vi "DHE_ParseCommand.vi"(0 "fd":i32, 1 "Log":bool=TRUE, 5 "command + args":string, 7 "command":string, 9 "arguments":string, 11 "error in":errorcluster, 12 "modpath":path) -> (4 "DHE_DBSRef":T1, 6 "message":string, 8 "OK message":string="DONE", 10 "TimeOut out":i32, 15 "error out":errorcluster)   [LabVIEW 2016]
uses:
  DBSHAND/private/vis/DatabaseHand_RefNum.ctl
  DHE_TP_action.ctl
  DBSHAND/private/vis/DatabaseHand_Element_Get(string).vi
  DBSHAND/private/vis/DatabaseHand_Element_Set(double).vi
  DBSHAND/private/vis/DatabaseHand_Element_Get(bool).vi
  DBSHAND/private/vis/DatabaseHand_Element_Get(double).vi
  DBSHAND/private/vis/DatabaseHand_Element_Get(I32).vi
  DBSHAND/private/vis/DatabaseHand_Element_Get(U32).vi
  DBSHAND/private/vis/DatabaseHand_Element_Set(string).vi
  DBSHAND/private/vis/DatabaseHand_Element_Set(2DArr).vi
  DBSHAND/private/vis/DatabaseHand_Element_Set(bool).vi
panel:
  in  "DHE_Aliasfile":path
  out "timeout offset":i32=20000
  in  "initimeout":i32=-1
  out "expscript":path
  in  "shutdownmacro":string
  in  "initmacro":string
  in  "extshut":bool
  in  "appendid":bool
  in  "expasync":bool=TRUE
  in  "artifpatterns":string
  in  "FPAreadmode":string
  in  "FPAmodifiers":string
  in  "FPAname":string
  in  "DHE_InstLib":path
  in  "DHE_REGfile":path
  in  "DHE_DACfile":path
  in  "DHE_Mod":string
  in  "log":bool
  in  "DHE_LogFile":path
  in  "DHE_MacroDir":path
  out "ConfigFile":path
  in  "Algors_file":path
  in  "TP_file":path
  in  "Init_file":path
  in  "Config":string[][](table)=[["INIT", "file", "DHE_ParseCommand.vi", "Init_file", "none", "PATH"], ["INIT", "module", "DHE_ParseCommand.vi", "DHE_Mod", "", "STR"], ["INIT", "initmacro", "DHE_ParseCommand.vi", "initmacro", "", "STR"], ["INIT", "timeout_s", "DHE_ParseCommand.vi", "initimeout", "", "I32"], ["TP", "tpfile", "DHE_ParseCommand.vi", "TP_file", "none", "PATH"], ["TP", "algorfile", "DHE_ParseCommand.vi", "Algors_file", "none", "PATH"], ["LOG", "file", "DHE_ParseCommand.vi", "DHE_LogFile", "none", "PATH"], ["LOG", "log", "DHE_ParseCommand.vi", "log", "FALSE", "BOOL"], ["MACROS", "dir", "DHE_ParseCommand.vi", "DHE_MacroDir", "", "PATH"], ["DACS", "file", "DHE_ParseCommand.vi", "DHE_DACfile", "", "PATH"], ["REGS", "file", "DHE_ParseCommand.vi", "DHE_REGfile", "", "PATH"], ["INSTLIB", "lib", "DHE_ParseCommand.vi", "DHE_InstLib", "", "PATH"], ["FPA", "name", "DHE_ParseCommand.vi", "FPAname", "", "STR"], ["FPA", "modifiers", "DHE_ParseCommand.vi", "FPAmodifiers", "", "STR"], ["FPA", "readmode", "DHE_ParseCommand.vi", "FPAreadmode", "", "STR"], ["ARTIF", "patterns", "DHE_ParseCommand.vi", "artifpatterns", "", "STR"], ["MISC", "appendid", "DHE_ParseCommand.vi", "appendid", "", "BOOL"], ["MISC", "expasync", "DHE_ParseCommand.vi", "expasync", "", "BOOL"], ["MISC", "shutdownmacro", "DHE_ParseCommand.vi", "shutdownmacro", "", "STR"], ["SHUTTER", "external", "DHE_ParseCommand.vi", "extshut", "", "BOOL"], ["ALIAS", "file", "DHE_ParseCommand.vi", "DHE_Aliasfile", "", "PATH"]]
  in  "ModuleName":string="DHE"
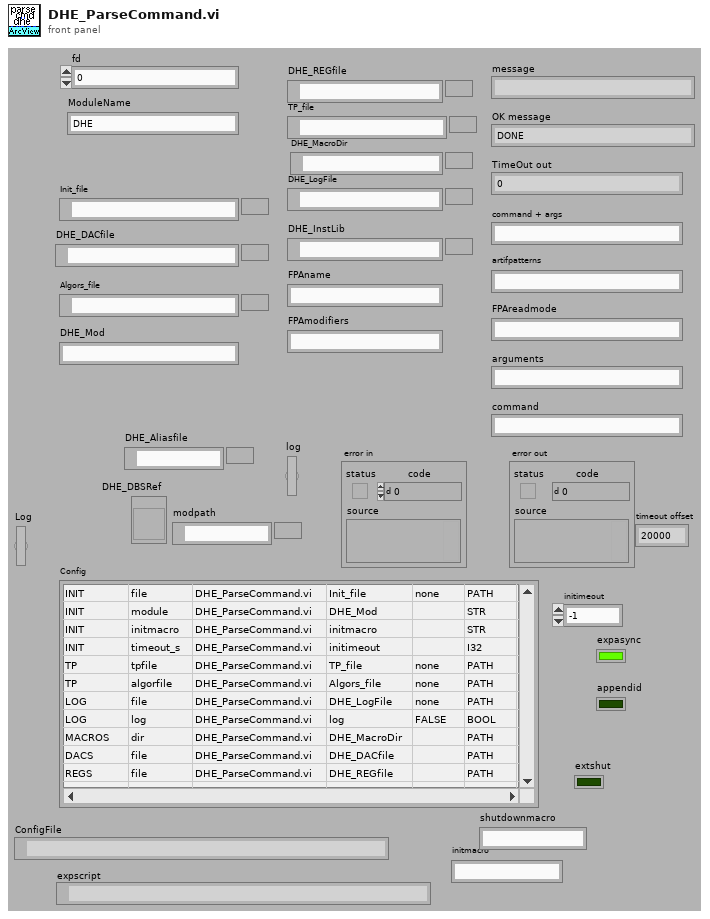
[diagram p1: front panel]
types:
  T1 = typedef "DatabaseHand_RefNum.ctl" = refnum<vi>
  T2 = enum16{"Idle", "Exposing", "Paused", "AbortExp", "Reading", "AbortRead", "FinishedReading", "Resetting", "Reducing", "Initializing"}
  T3 = enum16{"Idle", "Exposing", "Paused", "AbortExp", "Reading", "AbortRead", "FinishedReading"}
  T4 = enum16{"get fd", "set fd", "add ", "set_readtime", "get all", "clean all", "get by fd"}
  T5 = enum16{"get fd", "set fd", "add ", "set_readtime", "get all", "clean all"}
  T6 = typedef "DHE_TP_action.ctl" = enum16{"READ FROM FILE", "GET ALL", "FIND BY NAME", "FIND BY TYPE", "SET VALUE", "CLEAN", "CHANGE", "GET EXPUPDATE"}
  T7 = enum16{"read from file", "clear", "get all", "set all"}
  T8 = enum16{"get", "send", "delete", "add", "clean", "send_all", "send_on", "send_off", "use_stat", "use_async"}
  T9 = enum16{"read from file", "find", "get", "add", "delete", "clear "}
  T10 = typedef "DHE_Obs.ctl" = cluster{"observer":string, "obstype":string, "exptime":dbl, "coadds":i32, "fowler":i32, "nimages":i32, "display":bool, "autowrite":bool, "frames to write":cluster{"subs":bool, "reset":bool, "exposed":bool}, "frames to display":cluster{"subs":bool, "reset":bool, "exposed":bool}, "sur":i32}
  T11 = typedef "CMN_ContStatus.ctl" = cluster{"Response":string, "power":bool, "shutter":bool, "artifdata":bool, "idlemode":bool, "reset":bool, "gain":u8, "speed":u8, "resetPCI":bool, "autoshutter":bool, "TempSetPoint":i32, "multipleextensions":bool, "displayImage":bool, "coadding":bool, "images being coadded":i32, "Operation Mode":enum16{"normal", "coadd", "fawler"}, "frames to write":cluster{"subs":bool, "reset":bool, "exposed":bool}, "fawler samples":i32, "write auto":bool, "datatype":string, "frames to display":cluster{"subs":bool, "reset":bool, "exposed":bool}, "sur":i32, "autoclear":bool}
  T12 = typedef "DHE_Device.ctl" = cluster{"DevNo":i32, "fd":i32, "name":string, "FPA":string, "modifiers":string, "binpatt":string, "readtime":dbl, "readmode":string, "type":string, "params":string}
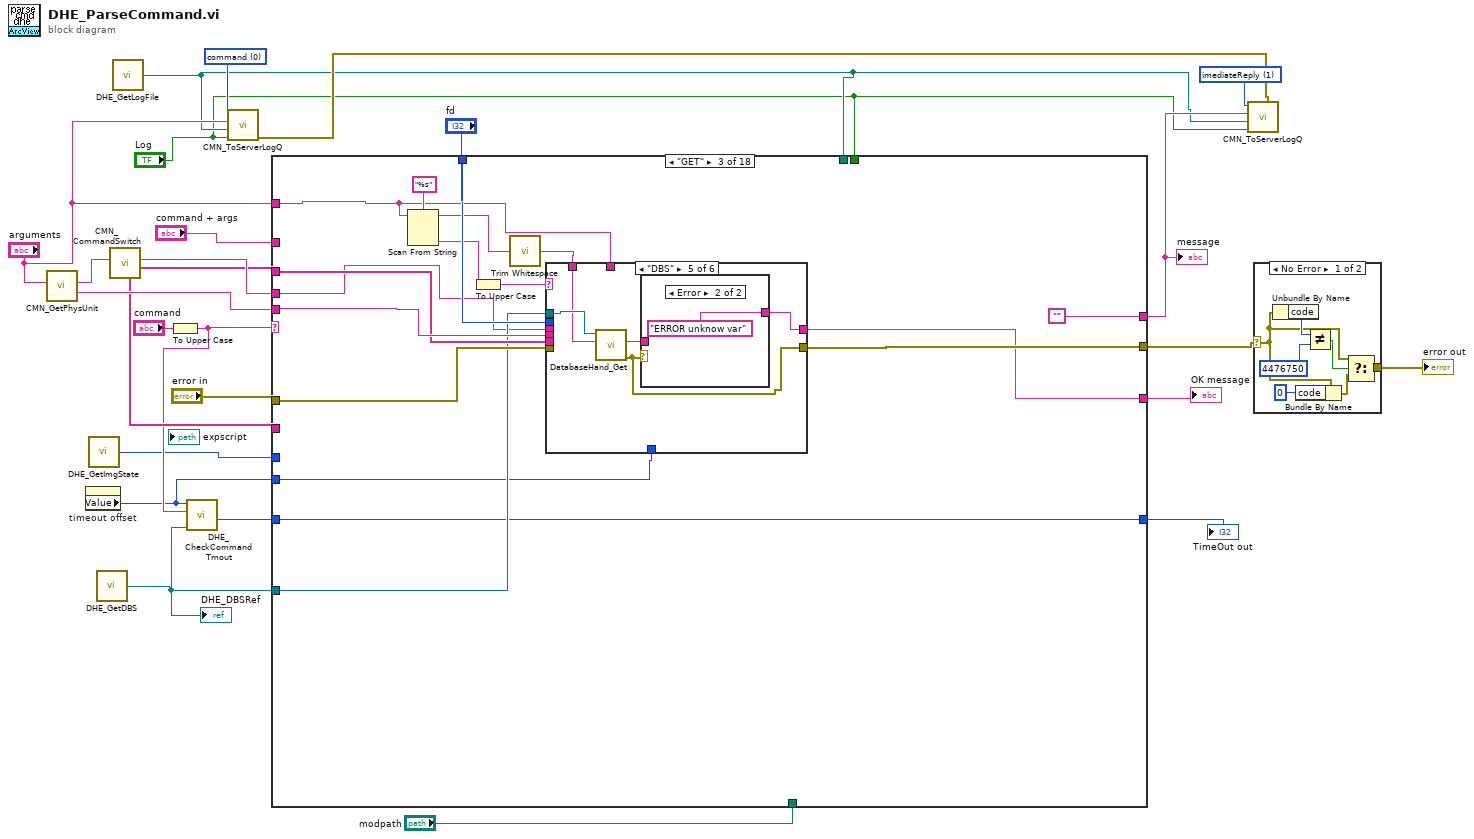
[diagram p0: block diagram]
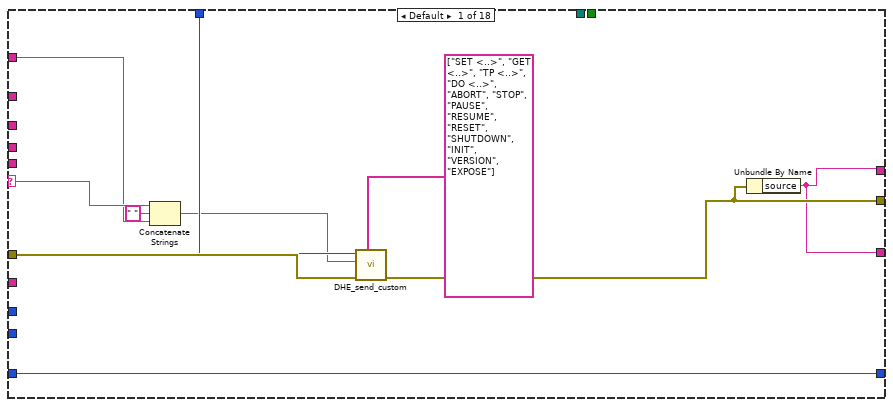
[diagram p3: hidden frame]
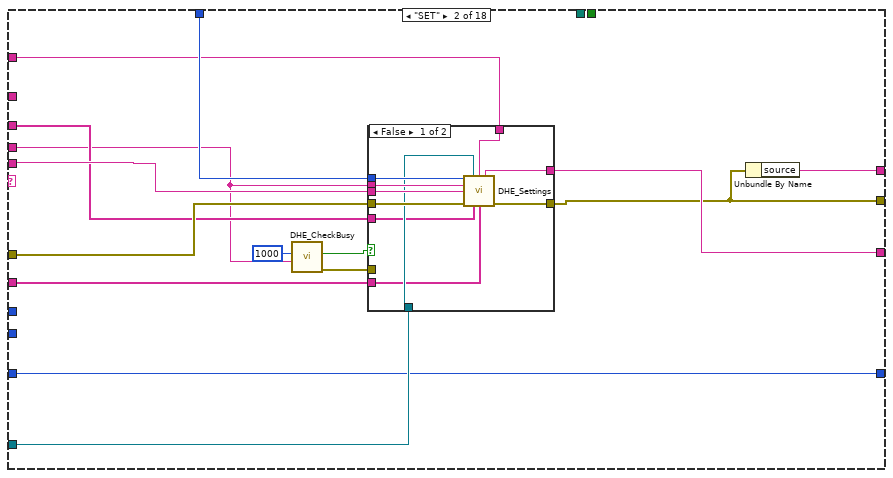
[diagram p4: hidden frame]
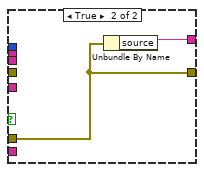
[diagram p5: hidden frame]
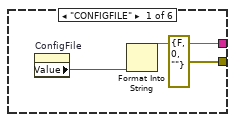
[diagram p6: hidden frame]
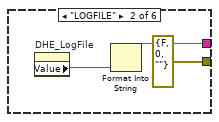
[diagram p7: hidden frame]
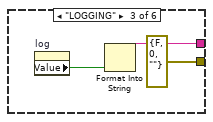
[diagram p8: hidden frame]
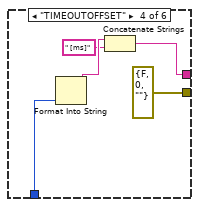
[diagram p9: hidden frame]
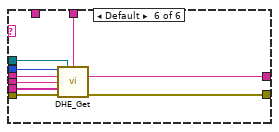
[diagram p11: hidden frame]
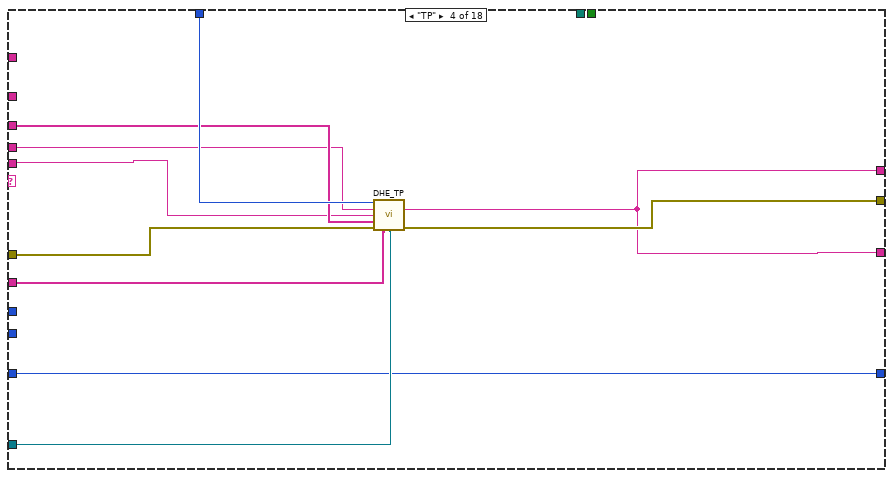
[diagram p12: hidden frame]
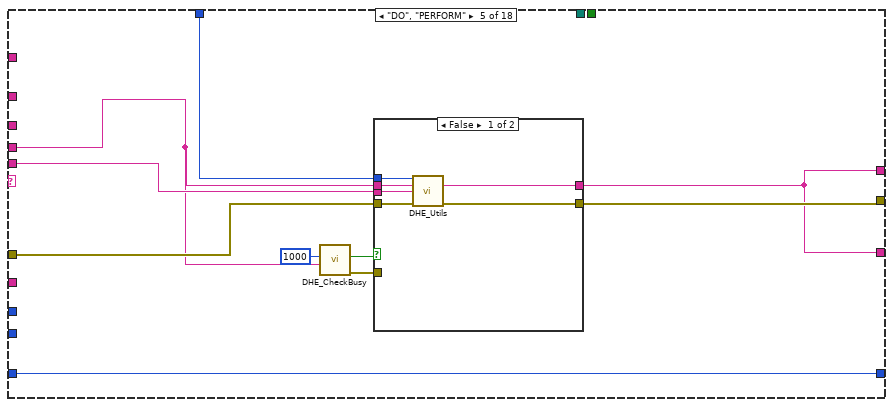
[diagram p13: hidden frame]
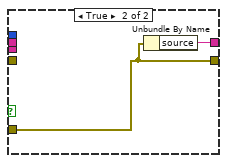
[diagram p14: hidden frame]
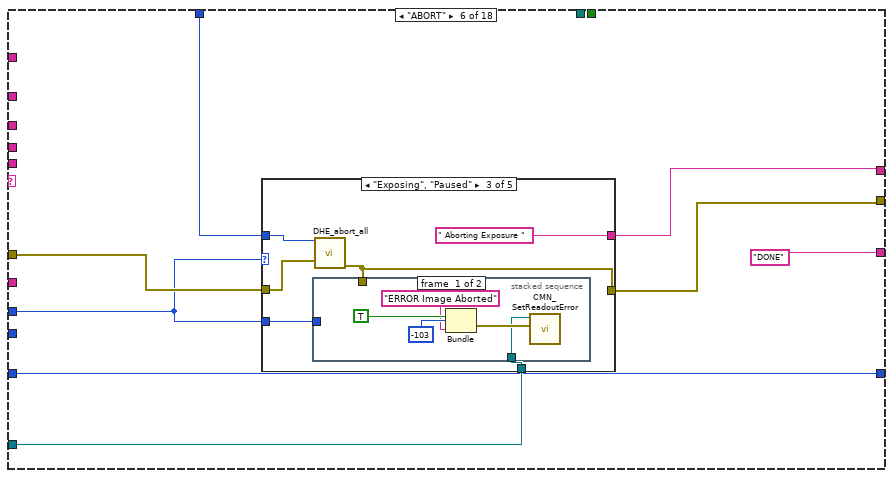
[diagram p15: hidden frame]
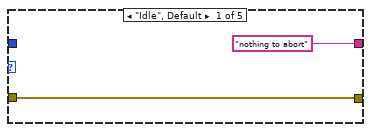
[diagram p16: hidden frame]
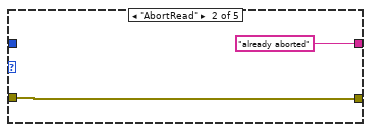
[diagram p17: hidden frame]
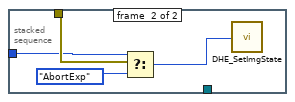
[diagram p18: hidden frame]
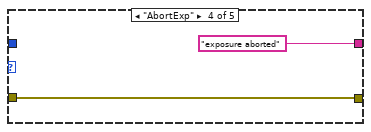
[diagram p19: hidden frame]
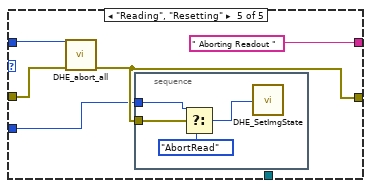
[diagram p20: hidden frame]
diagram:
  w6 = u16 1 items=["command", "imediateReply", "Callback Reply", "Information"] ("type")
  w8 = u16 0 items=["command", "imediateReply", "Callback Reply", "Information"] ("type")
  n1 = call "CMN_GetPhysUnit.vi"("command in"="arguments") -> ("unit"=w23:string, "command out"=w21:string)  [unwired: 9 out]
  n2 = property on="timeout offset" class="DigNum (strict)"() -> ("Value"=w1:i32)  [unwired: 2 in, 2 out]
  n3 = call "DHE_GetImgState.vi"() -> ("DHE_ImgState"=w12:T2)  [unwired: 9 out]
  n4 = call "DHE_GetDBS.vi"() -> ("DHE_DBSRef"=w13:T1)  [unwired: 9 out]
  "DHE_DBSRef" <- w13
  n5 = call "CMN_CommandSwitch.vi"("command in"=w21) -> ("swhitches"=w19:string[], "command out"=w20:string, "arguments"=w18:string[])  [unwired: 1 in, 7 out]
  n6 = call "DHE_GetLogFile.vi"() -> ("DHE_LogFile"=w3:path)  [unwired: 9 out]
  n7 = To Upper Case(1:"command") -> (0:w16:string)
  n8 = call "DHE_CheckCommandTmout.vi"("DBSRef"=w13, "Command"=w16, "TimeOut in"=w1) -> ("TimeOut out"=w11:i32)  [unwired: 2 in, 5 out]
  n9 = call "CMN_ToServerLogQ.vi"("Log"="Log", "file"=w3, "string"="arguments", "type"=w8) -> ("error out"=w4:errorcluster)  [unwired: 2 in, 4 out]
  n10 = case shown="\"GET\"" w16 {
    selector: w16 -> [w32 _ _ _ _ _ _ _ _ _ _ _ _ _ _ _ _ _]
    tunnel: "error in" -> [w36 w51 w80 w120 w130 w145 w189 w294 w332 w340 w369 w397 w462 w516 w669 w796 _ _]
    tunnel: [w35 w46 w79 w118 w129 w144 w188 w296 w332 w335 w364 w396 w446 w514 w669 w794 errorcluster {"status"=FALSE, "code"=0, "source"=""} ("error out") errorcluster {"status"=FALSE, "code"=0, "source"=""} ("error out")] -> w15
    tunnel: w20 -> [_ w37 w70 w113 w121 _ w187 _ _ _ _ w401 _ w526 w670 _ w801 w817]
    tunnel: "fd" -> [w33 w50 w78 w119 w128 w146 w182 w295 _ w339 w368 w398 w448 _ _ w793 _ _]
    tunnel: [w34 w45 "" w115 w126 w143 w177 w290 w331 w338 w367 w395 "Closing Controller" w517 "async" ("SDSDUII ModuleName") w789 w803 w819] -> w5
    tunnel: "command + args" -> [_ _ _ _ _ _ _ _ _ _ _ _ _ _ _ _ _ _]
    tunnel: w23 -> [_ w49 w76 w114 w127 _ _ _ _ _ _ _ _ _ _ _ _ _]
    tunnel: [w34 w47 w75 w115 w126 "DONE" "DONE" w284 w331 "DONE" "DONE" "DONE" "DONE" w511 w667 w789 w803 w819] -> w22
    tunnel: w19 -> [_ w43 w74 w116 _ _ _ _ _ _ _ _ _ w504 _ w800 _ _]
    tunnel: w18 -> [_ w42 _ w117 _ _ _ _ _ _ _ _ _ _ _ _ _ _]
    tunnel: w13 -> [_ w44 w73 w112 _ w140 w181 w280 w327 w333 w362 _ w461 _ w674 _ _ w816]
    tunnel: w12 -> [_ _ _ _ _ w141 w183 _ _ w336 w365 _ _ _ _ _ _ _]
    tunnel: "arguments" -> [w27 w39 w65 _ _ _ _ _ _ _ _ w391 _ _ _ _ _ _]
    tunnel: w11 -> [w30 w40 w72 w111 w125 w139 w180 w291 _ w334 w363 w393 w444 w501 w673 w787 w807 w823]
    tunnel: [w30 w40 w72 w111 w125 w139 w180 w291 w330 w334 w363 w393 w444 w500 w673 w787 w807 w823] -> w10
    tunnel: "modpath" -> [_ _ _ _ _ _ _ _ _ _ _ _ _ w505 _ _ _ _]
    tunnel: w3 -> [_ _ _ _ _ _ _ _ _ _ _ _ _ w503 _ _ _ _]
    tunnel: "Log" -> [_ _ _ _ _ _ _ _ _ _ _ _ _ w502 _ _ _ _]
    tunnel: w1 -> [_ _ w71 _ _ _ _ _ _ _ _ _ _ _ _ _ _ _]
    frame Default {
      n11 = Concatenate Strings(w32, " " ("string"), w27) -> (w29:string)
      n12 = call "DHE_send_custom.vi"("valid params"=string[] ["SET <..>", "GET <..>", "TP <..>", "DO <..>", "ABORT", "STOP", "PAUSE", "RESUME", "RESET", "SHUTDOWN", "INIT", "VERSION", "EXPOSE"], "error in (no error)"=w36, "args"=w29, "fd"=w33) -> ("error IO"=w35:errorcluster)  [unwired: 7 out]
      n13 = Unbundle By Name(w35) -> ("source"=w34:string)
    }
    frame "SET" {
      n14 = call "DHE_CheckBusy.vi"("command"=w37, "timeout (2000 ms)"=u32 1000) -> ("error out"=w48:errorcluster, "busy?"=w41:bool)  [unwired: 1 in, 7 out]
      n15 = case shown="False" w41 {
        tunnel: w51 -> [w61 _]
        tunnel: [w60 w63] -> w46
        tunnel: w50 -> [w59 _]
        tunnel: w37 -> [w58 _]
        tunnel: w49 -> [w57 _]
        tunnel: w48 -> [_ w63]
        tunnel: [w56 w62] -> w47
        tunnel: w44 -> [w55 _]
        tunnel: w43 -> [w54 _]
        tunnel: w42 -> [w53 _]
        tunnel: w39 -> [w52 _]
        frame False {
          n16 = call "DHE_Settings.vi"("refnum"=w59, "DHE_DBSRef"=w55, "raw args"=w52, "Command"=w58, "physical unit"=w57, "error in (no error)"=w61, "switches"=w54, "switches args"=w53) -> ("message"=w56:string, "error out"=w60:errorcluster)  [unwired: 6 out]
        }
        frame True {
          n17 = Unbundle By Name(w63) -> ("source"=w62:string)
        }
      }
      n18 = Unbundle By Name(w46) -> ("source"=w45:string)
    }
    frame "GET" {
      n19 = Scan From String(format string="%s", input string=w65) -> (remaining string=w67:string, output 1=w68:string)  [unwired: 3 in, 2 out]
      n20 = To Upper Case(1:w68) -> (0:w64:string)
      n21 = call <vilib>:"Trim Whitespace.vi"("string"=w67) -> ("trimmed string"=w66:string)  [unwired: 1 in]
      n22 = case shown="\"DBS\"" w64 {
        tunnel: w80 -> [_ _ _ _ _ w110]
        tunnel: [errorcluster {"status"=FALSE, "code"=0, "source"=""} ("error out") errorcluster {"status"=FALSE, "code"=0, "source"=""} ("error out") errorcluster {"status"=FALSE, "code"=0, "source"=""} ("error out") errorcluster {"status"=FALSE, "code"=0, "source"=""} ("error out") w97 w109] -> w79
        tunnel: w78 -> [_ _ _ _ _ w108]
        tunnel: w70 -> [_ _ _ _ _ w107]
        tunnel: w76 -> [_ _ _ _ _ w106]
        tunnel: [w82 w86 w89 w91 w96 w105] -> w75
        tunnel: w74 -> [_ _ _ _ _ w104]
        tunnel: w73 -> [_ _ _ _ w98 w103]
        tunnel: w65 -> [_ _ _ _ _ w102]
        tunnel: w71 -> [_ _ _ w93 _ _]
        tunnel: w66 -> [_ _ _ _ w95 _]
        frame "CONFIGFILE" {
          n23 = property on="ConfigFile" class="Path"() -> ("Value"=w83:path)  [unwired: 2 in, 2 out]
          n24 = Format Into String(w83) -> (resulting string=w82:string)  [unwired: 3 in, 1 out]
        }
        frame "LOGFILE" {
          n25 = property on="DHE_LogFile" class="Path"() -> ("Value"=w84:path)  [unwired: 2 in, 2 out]
          n26 = Format Into String(w84) -> (resulting string=w86:string)  [unwired: 3 in, 1 out]
        }
        frame "LOGGING" {
          n27 = property on="log" class="Bool (strict)"() -> ("Value"=w87:bool)  [unwired: 2 in, 2 out]
          n28 = Format Into String(w87) -> (resulting string=w89:string)  [unwired: 3 in, 1 out]
        }
        frame "TIMEOUTOFFSET" {
          n29 = Format Into String(w93) -> (resulting string=w92:string)  [unwired: 3 in, 1 out]
          n30 = Concatenate Strings(w92, " [ms]" ("string")) -> (w91:string)
        }
        frame "DBS" {
          n31 = call-poly "DatabaseHand_Get.vi"("name"=w95, "Database RefNum in"=w98) -> ("error out"=w97:errorcluster, "value"=w99:string)  [unwired: 3 in, 5 out]
          n32 = case shown="Error" w97 {
            tunnel: [w100 "ERROR unknow var" ("response")] -> w96
            tunnel: w99 -> [w100 _]
            frame No Error {
            }
            frame Error {
            }
          }
        }
        frame Default {
          n33 = call "DHE_Get.vi"("refnum"=w108, "DHE_DBSRef"=w103, "Command + switches"=w102, "Command"=w107, "physical unit"=w106, "swhitches"=w104, "error in (no error)"=w110) -> ("response"=w105:string, "error out"=w109:errorcluster)  [unwired: 7 out]
        }
      }
    }
    frame "TP" {
      n34 = call "DHE_TP.vi"("refnum"=w119, "Command"=w113, "physical unit"=w114, "swhitches"=w116, "error in (no error)"=w120, "switch arguments"=w117, "Database RefNum in"=w112) -> ("response"=w115:string, "error out"=w118:errorcluster)  [unwired: 7 out]
    }
    frame "DO", "PERFORM" {
      n35 = call "DHE_CheckBusy.vi"("command"=w121, "timeout (2000 ms)"=u32 1000) -> ("error out"=w122:errorcluster, "busy?"=w123:bool)  [unwired: 1 in, 7 out]
      n36 = case shown="False" w123 {
        tunnel: w130 -> [w136 _]
        tunnel: [w135 w138] -> w129
        tunnel: w128 -> [w134 _]
        tunnel: w127 -> [w133 _]
        tunnel: w121 -> [w132 _]
        tunnel: [w131 w137] -> w126
        tunnel: w122 -> [_ w138]
        frame False {
          n37 = call "DHE_Utils.vi"("refnum"=w134, "Command"=w132, "physical unit"=w133, "error in (no error)"=w136) -> ("message"=w131:string, "error out"=w135:errorcluster)  [unwired: 10 out]
        }
        frame True {
          n38 = Unbundle By Name(w138) -> ("source"=w137:string)
        }
      }
    }
    frame "ABORT" {
      n39 = case shown="\"Exposing\", \"Paused\"" w141 {
        tunnel: w146 -> [_ _ w153 _ w171]
        tunnel: w145 -> [w147 w150 w155 w167 w170]
        tunnel: [w147 w150 w154 w167 w169] -> w144
        tunnel: ["nothing to abort" "already aborted" " Aborting Exposure " "exposure aborted" " Aborting Readout "] -> w143
        tunnel: w141 -> [_ _ w152 _ w168]
        tunnel: w140 -> [_ _ w151 _ _]
        frame "Idle", Default {
        }
        frame "AbortRead" {
        }
        frame "Exposing", "Paused" {
          n40 = call "DHE_abort_all.vi"("fd"=w153, "error in (no error)"=w155) -> ("error out"=w154:errorcluster)  [unwired: 13 out]
          n41 = stacked-sequence {
            tunnel: w154 -> [_ w165]
            tunnel: w152 -> [_ w163]
            tunnel: w151 -> [w157 _]
            frame #0 {
              n42 = Bundle(TRUE, -103, "ERROR Image Aborted") -> (w158:errorcluster)  [unwired: 1 out]
              n43 = call "CMN_SetReadoutError.vi"("readout error"=w158, "Database RefNum in"=w157) -> ()  [unwired: 1 in, 9 out]
            }
            frame #1 {
              n44 = Select(t=w163, s=w165, f=T3."AbortExp" ("ImgState")) -> (s? t:f=w162:T2)
              n45 = call "DHE_SetImgState.vi"("DHE_ImgState"=w162) -> ()  [unwired: 9 out]
            }
          }
        }
        frame "AbortExp" {
        }
        frame "Reading", "Resetting" {
          n46 = call "DHE_abort_all.vi"("fd"=w171, "error in (no error)"=w170) -> ("error out"=w169:errorcluster)  [unwired: 13 out]
          n47 = stacked-sequence {
            tunnel: w169 -> [w176]
            tunnel: w168 -> [w174]
            frame #0 {
              n48 = Select(t=w174, s=w176, f=T3."AbortRead" ("ImgState")) -> (s? t:f=w173:T2)
              n49 = call "DHE_SetImgState.vi"("DHE_ImgState"=w173) -> ()  [unwired: 9 out]
            }
          }
        }
      }
    }
    frame "STOP" {
      n50 = Scan From String(format string="%s" ("Format String"), input string=w187) -> (remaining string=w179:string, output 1=w185:string)  [unwired: 2 in, 3 out]
      n51 = To Lower Case(string=w185) -> (all lower case string=w184:string)
      n52 = case shown="\"sur\"" w184 {
        tunnel: w189 -> [w192 w208 w233 w250 w267]
        tunnel: [w194 w210 w235 w252 w269] -> w188
        tunnel: w183 -> [w193 w209 w234 w251 w268]
        tunnel: w182 -> [w191 w207 w232 w249 w266]
        tunnel: w181 -> [_ w206 w231 w248 w265]
        tunnel: w179 -> [_ w205 w230 w247 w264]
        tunnel: [w190 w204 w229 w246 w263] -> w177
        frame "sequence", Default {
          n53 = case shown="Default" w193 {
            tunnel: w192 -> [w199 w202]
            tunnel: [w198 w203] -> w194
            tunnel: w191 -> [_ w201]
            tunnel: [w195 "DONE"] -> w190
            frame "Idle" {
              w195 = "STOP SEQ: nothing to stop" ("source")
              n54 = Bundle By Name(cluster=w199, "status"=FALSE, "code"=-1, "source"=w195) -> (w198:errorcluster)
            }
            frame Default {
              n55 = call "DHE_stop_sequence.vi"("fd in"=w201, "error in (no error)"=w202) -> ("error out"=w203:errorcluster)  [unwired: 13 out]
            }
          }
        }
        frame "exp", "exposure" {
          n56 = case shown="\"Exposing\"..\"AbortExp\"" w209 {
            tunnel: w208 -> [w215 w220]
            tunnel: [w214 w219] -> w210
            tunnel: w207 -> [_ w222]
            tunnel: w206 -> [_ w217]
            tunnel: w205 -> [_ w221]
            tunnel: [w211 "DONE"] -> w204
            frame Default {
              w211 = "STOP EXP: nothing to stop" ("source")
              n57 = Bundle By Name(cluster=w215, "status"=FALSE, "code"=-1, "source"=w211) -> (w214:errorcluster)
            }
            frame "Exposing".."AbortExp" {
              n58 = call "DHE_Stop.vi"("DHE_DBSRef"=w217, "error in (no error)"=w220, "args"=w221, "fd"=w222) -> ("error out"=w219:errorcluster, "return value"=w218:i32)  [unwired: 6 out]
              n59 = case shown="No Error" w219 {
                tunnel: w217 -> [w228 _]
                tunnel: w218 -> [w225 _]
                frame No Error {
                  # "sets the actual\nexposure time when it\nwas stoped"
                  n60 = Divide(x=w225, y=1000) -> (x/y=w223:dbl)
                  n61 = call-poly "DatabaseHand_Set.vi"("group"="obs", "name"="aexptime", "value"=w223, "Database RefNum in"=w228) -> ()  [unwired: 4 in, 4 out]
                }
                frame Error {
                }
              }
            }
          }
        }
        frame "coadd", "coadding", "coadds" {
          n62 = case shown="Default" w234 {
            tunnel: w233 -> [w240 _]
            tunnel: [w239 w242] -> w235
            tunnel: w232 -> [_ w245]
            tunnel: w231 -> [_ _]
            tunnel: w230 -> [_ _]
            tunnel: [w236 w243] -> w229
            frame "Idle" {
              w236 = "STOP EXP: nothing to stop" ("source")
              n63 = Bundle By Name(cluster=w240, "status"=FALSE, "code"=-1, "source"=w236) -> (w239:errorcluster)
            }
            frame Default {
              n64 = call "DHE_stop_coadds.vi"("fd"=w245) -> ("error out"=w242:errorcluster)  [unwired: 1 in, 13 out]
              n65 = Unbundle By Name(w242) -> ("source"=w241:string)
              n66 = Select(t=w241, s=w242, f="DONE" ("SDSDUII ModuleName")) -> (s? t:f=w243:string)
            }
          }
        }
        frame "all", "now" {
          n67 = case shown="Default" w251 {
            tunnel: w250 -> [w257 _]
            tunnel: [w256 w259] -> w252
            tunnel: w249 -> [_ w262]
            tunnel: w248 -> [_ _]
            tunnel: w247 -> [_ _]
            tunnel: [w253 w260] -> w246
            frame "Idle" {
              w253 = "STOP ALL: nothing to stop" ("source")
              n68 = Bundle By Name(cluster=w257, "status"=FALSE, "code"=-1, "source"=w253) -> (w256:errorcluster)
            }
            frame Default {
              n69 = call "DHE_stop_all.vi"("fd"=w262) -> ("error out"=w259:errorcluster)  [unwired: 1 in, 13 out]
              n70 = Unbundle By Name(w259) -> ("source"=w258:string)
              n71 = Select(t=w258, s=w259, f="DONE" ("SDSDUII ModuleName")) -> (s? t:f=w260:string)
            }
          }
        }
        frame "sur" {
          n72 = case shown="Default" w268 {
            tunnel: w267 -> [w274 _]
            tunnel: [w273 w276] -> w269
            tunnel: w266 -> [_ w279]
            tunnel: w265 -> [_ _]
            tunnel: w264 -> [_ _]
            tunnel: [w270 w277] -> w263
            frame "Idle" {
              w270 = "STOP EXP: nothing to stop" ("source")
              n73 = Bundle By Name(cluster=w274, "status"=FALSE, "code"=-1, "source"=w270) -> (w273:errorcluster)
            }
            frame Default {
              n74 = call "DHE_stop_sur.vi"("fd"=w279) -> ("error out"=w276:errorcluster)  [unwired: 1 in, 13 out]
              n75 = Unbundle By Name(w276) -> ("source"=w275:string)
              n76 = Select(t=w275, s=w276, f="DONE" ("SDSDUII ModuleName")) -> (s? t:f=w277:string)
            }
          }
        }
      }
    }
    frame "EXPOSE" {
      n77 = call-poly "DatabaseHand_Get.vi"("default value"=TRUE, "name"="chkinterlock", "Database RefNum in"=w280) -> ("value"=w281:bool)  [unwired: 2 in, 6 out]
      n78 = case shown="True" w281 {
        tunnel: w294 -> [w297 w301]
        tunnel: [w297 w300] -> w293
        tunnel: [FALSE ("busy?") w299] -> w292
        frame False {
        }
        frame True {
          n79 = call "DHE_CheckBusy.vi"("error in (no error)"=w301) -> ("error out"=w300:errorcluster, "busy?"=w299:bool)  [unwired: 2 in, 7 out]
        }
      }
      n80 = case shown="False" w292 {
        tunnel: [w304 w316] -> w296
        tunnel: w295 -> [w306 _]
        tunnel: w293 -> [w305 w316]
        tunnel: [w302 w315] -> w286
        tunnel: w291 -> [w303 _]
        tunnel: [w302 w315] -> w290
        frame False {
          n81 = call "DHE_Expose.vi"("error in"=w305, "fd"=w306) -> ("error out"=w304:errorcluster)  [unwired: 2 out]
          n82 = case shown="No Error" w304 {
            selector: w304 -> [_ w314]
            tunnel: [w308 w311] -> w302
            tunnel: w303 -> [w307 _]
            frame No Error {
              n83 = Format Into String(format string="%s %d", "OK", w307) -> (resulting string=w308:string)  [unwired: 2 in, 1 out]
            }
            frame Error {
              n84 = Unbundle By Name(w314) -> ("source"=w313:string)
              n85 = Concatenate Strings("ERROR " ("string"), w313) -> (w311:string)
            }
          }
        }
        frame True {
          n86 = Unbundle By Name(w316) -> ("source"=w315:string)
        }
      }
      n87 = call-poly "DatabaseHand_Get.vi"("default value"=FALSE, "name"="armed", "Database RefNum in"=w280) -> ("value"=w287:bool)  [unwired: 2 in, 6 out]
      n88 = Select(t="READY", s=w287, f=w286) -> (s? t:f=w284:string)
    }
    frame "INTEGRATE" {
      n89 = call "DHE_GetObsParams.vi"() -> ("DHE_OBS"=w325:T10)  [unwired: 11 out]
      n90 = Unbundle By Name(w325) -> ("exptime"=w321:dbl)
      n91 = call-poly "DatabaseHand_Get.vi"("default value"=w321, "name"="rintegtime", "Database RefNum in"=w327) -> ("value"=w320:dbl)  [unwired: 2 in, 6 out]
      n92 = Greater Or Equal To 0?(x=w320) -> (x >= 0?=w322:bool)
      n93 = Select(t=w320, s=w322, f=w321) -> (s? t:f=w319:dbl)
      n94 = Add(x=w319, y=5.0) -> (x+y=w317:dbl)
      n95 = Multiply(x=w317, y=u32 1000) -> (x*y=w328:dbl)
      n96 = To Unsigned Long Integer(number=w328) -> (unsigned 32bit integer=w330:u32)
      n97 = Format Into String(format string="%s %d", "OK", w330) -> (resulting string=w331:string)  [unwired: 2 in, 1 out]
    }
    frame "PAUSE" {
      n98 = case shown="\"Exposing\"" w336 {
        tunnel: w340 -> [w344 w353]
        tunnel: w339 -> [_ w347]
        tunnel: [w343 w351] -> w335
        tunnel: [w342 "Pausing Exposure" ("trimmed string")] -> w338
        tunnel: w333 -> [_ w348]
        frame "Idle", Default {
          w342 = "Pause Exposure: Not Exposing"
          n99 = Bundle By Name(cluster=w344, "status"=TRUE, "code"=-1, "source"=w342) -> (w343:errorcluster)
        }
        frame "Exposing" {
          n100 = call-poly "DatabaseHand_Get.vi"("default value"=FALSE, "name"="local_integ", "Database RefNum in"=w348) -> ("value"=w346:bool)  [unwired: 2 in, 6 out]
          n101 = case shown="True" w346 {
            tunnel: w353 -> [w356 _]
            tunnel: [w355 w358] -> w351
            tunnel: w347 -> [w354 w360]
            frame False {
              n102 = call "DHE_pause_exposure.vi"("fd"=w354, "error in (no error)"=w356) -> ("error out"=w355:errorcluster)  [unwired: 13 out]
            }
            frame True {
              n103 = call "DHE_move_shutter.vi"("fd"=w360, "flag"=i16 0) -> ("error out"=w358:errorcluster)  [unwired: 1 in, 12 out]
              n104 = call "DHE_Lib_pause_integrate.vi"("error in (no error)"=w358) -> ("error out"=w357:errorcluster)  [unwired: 14 out]
              n105 = case shown="No Error" w357 {
                frame No Error {
                  n106 = call "DHE_SetImgState.vi"("DHE_ImgState"=T2."Paused") -> ()  [unwired: 9 out]
                }
                frame Error {
                }
              }
            }
          }
        }
      }
    }
    frame "RESUME" {
      n107 = case shown="\"Paused\"" w365 {
        tunnel: w369 -> [w373 w382]
        tunnel: w368 -> [_ w381]
        tunnel: [w372 w379] -> w364
        tunnel: [w370 "Resuming Exposure" ("trimmed string")] -> w367
        tunnel: w362 -> [_ w376]
        frame "Idle", Default {
          w370 = "Resuming: Not Paused"
          n108 = Bundle By Name(cluster=w373, "status"=TRUE, "code"=-1, "source"=w370) -> (w372:errorcluster)
        }
        frame "Paused" {
          n109 = call-poly "DatabaseHand_Get.vi"("default value"=FALSE, "name"="local_integ", "Database RefNum in"=w376) -> ("value"=w375:bool)  [unwired: 2 in, 6 out]
          n110 = case shown="True" w375 {
            tunnel: w382 -> [w385 _]
            tunnel: w381 -> [w384 w389]
            tunnel: [w383 w386] -> w379
            frame False {
              n111 = call "DHE_resume_exposure.vi"("fd"=w384, "error in (no error)"=w385) -> ("error out"=w383:errorcluster)  [unwired: 13 out]
            }
            frame True {
              n112 = call "DHE_move_shutter.vi"("fd"=w389, "flag"=i16 1) -> ("error out"=w387:errorcluster)  [unwired: 1 in, 12 out]
              n113 = call "DHE_Lib_resume_integrate.vi"("error in (no error)"=w387) -> ("error out"=w386:errorcluster)  [unwired: 14 out]
              n114 = case shown="No Error" w386 {
                frame No Error {
                  n115 = call "DHE_SetImgState.vi"("DHE_ImgState"=T2."Exposing") -> ()  [unwired: 9 out]
                }
                frame Error {
                }
              }
            }
          }
        }
      }
    }
    frame "RESET" {
      n116 = Scan From String(format string="%s" ("Format String"), input string=w401) -> (remaining string=w392:string, output 1=w400:string)  [unwired: 2 in, 3 out]
      n117 = To Lower Case(string=w400) -> (all lower case string=w399:string)
      n118 = case shown="\"link\"" w399 {
        tunnel: w398 -> [w407 w413 w419 w425]
        tunnel: w397 -> [w404 w412 w418 w424]
        tunnel: [w405 w411 w417 w423] -> w396
        tunnel: [w406 "Resetting controller" "Resetting pci (computer)" "Resetting link (channel)"] -> w395
        tunnel: w392 -> [_ w409 w415 w421]
        tunnel: w391 -> [w403 _ _ _]
        frame Default {
          n119 = call "DHE_send_custom.vi"("error in (no error)"=w404, "args"=w403, "fd"=w407) -> ("error IO"=w405:errorcluster, "str result"=w406:string)  [unwired: 1 in, 6 out]
        }
        frame "controller" {
          n120 = call <vilib>:"Trim Whitespace.vi"("string"=w409) -> ("trimmed string"=w408:string)  [unwired: 1 in]
          n121 = call "DHE_reset_controller.vi"("fd"=w413, "arguments"=w408, "error in (no error)"=w412) -> ("error out"=w411:errorcluster)  [unwired: 12 out]
        }
        frame "pci" {
          n122 = call <vilib>:"Trim Whitespace.vi"("string"=w415) -> ("trimmed string"=w414:string)  [unwired: 1 in]
          n123 = call "DHE_reset_pci.vi"("fd"=w419, "arguments"=w414, "error in (no error)"=w418) -> ("error out"=w417:errorcluster)  [unwired: 12 out]
        }
        frame "link" {
          n124 = call <vilib>:"Trim Whitespace.vi"("string"=w421) -> ("trimmed string"=w420:string)  [unwired: 1 in]
          n125 = call "DHE_reset_link.vi"("fd"=w425, "arguments"=w420, "error in (no error)"=w424) -> ("error out"=w423:errorcluster)  [unwired: 12 out]
        }
      }
    }
    frame "CLOSE", "OFFLINE", "SHUTDOWN" {
      n126 = call "DHE_GetControllerStatus.vi"() -> ("ControllerStatus"=w466:T11)  [unwired: 11 out]
      n127 = call "DHE_TP.vi"("refnum"=w448, "Command"="DELETE", "error in (no error)"=w462) -> ("refnum out"=w463:i32)  [unwired: 4 in, 8 out]
      n128 = call-poly "DatabaseHand_Get.vi"("name"="basename", "Database RefNum in"=w461) -> ("value"=w452:string, "Database RefNum out"=w457:T1)  [unwired: 3 in, 5 out]
      n129 = Unbundle By Name(w466) -> ("power"=w467:bool)
      n130 = call-poly "DatabaseHand_Get.vi"("name"="imdir", "Database RefNum in"=w457) -> ("value"=w453:string, "Database RefNum out"=w456:T1)  [unwired: 3 in, 5 out]
      n131 = case shown="False" w467 {
        tunnel: w462 -> [w495 w499]
        tunnel: [w495 w498] -> _
        tunnel: w463 -> [w494 w496]
        tunnel: [w494 w496] -> w447
        frame False {
        }
        frame True {
          # "power off before closing"
          n132 = call "DHE_Utils.vi"("refnum"=w496, "Command"="power off", "error in (no error)"=w499) -> ("error out"=w498:errorcluster)  [unwired: 1 in, 11 out]
        }
      }
      n133 = call-poly "DatabaseHand_Get.vi"("default value"=1, "name"="imnumber", "Database RefNum in"=w456) -> ("value"=w454:i32, "Database RefNum out"=w451:T1)  [unwired: 2 in, 5 out]
      n134 = call-poly "DatabaseHand_Get.vi"("name"="froot", "Database RefNum in"=w451) -> ("value"=w449:string, "Database RefNum out"=w443:T1)  [unwired: 3 in, 5 out]
      n135 = call-poly "DatabaseHand_Get.vi"("name"="imprefix", "Database RefNum in"=w443) -> ("value"=w438:string, "Database RefNum out"=w442:T1)  [unwired: 3 in, 5 out]
      n136 = call "DHE_close_driver.vi"("fd"=w447) -> ("error out"=w446:errorcluster)  [unwired: 1 in, 13 out]
      n137 = Unbundle By Name(w446) -> ("code"=w445:i32)
      n138 = call-poly "DatabaseHand_Get.vi"("name"="imsufix", "Database RefNum in"=w442) -> ("value"=w439:string, "Database RefNum out"=w436:T1)  [unwired: 3 in, 5 out]
      n139 = case shown="-22, -9, 0" w445 {
        tunnel: w448 -> [w491 _]
        tunnel: w443 -> [w483 _]
        frame -22, -9, 0 {
          n140 = Number To Decimal String(number=w491) -> (decimal integer string=w490:string)  [unwired: 1 out]
          n141 = call-poly "DatabaseHand_Set.vi"("name"="dhe_firmware", "value"="_none_", "Database RefNum in"=w483) -> ()  [unwired: 5 in, 4 out]
          n142 = call "DHE_fdMgr.vi"("arg in"=w490, "action"=T4."get by fd") -> ("Device"=w488:T12)  [unwired: 3 in, 6 out]
          n143 = Unbundle By Name(w488) -> ("name"=w487:string)
          n144 = call "DHE_GetModRef.vi"() -> ("DHE_ModRef"=w485:refnum<vi>)  [unwired: 9 out]
          n145 = call "DHE_TP.vi"("Command"="delete") -> ()  [unwired: 6 in, 9 out]
          n146 = call "DHE_fdMgr.vi"("arg in"="0", "action"=T5."set fd", "cmd in"=w487) -> ()  [unwired: 2 in, 7 out]
          n147 = call "DHE_SetStatus.vi"("DHE_Status"="NOT INITIALIZED") -> ()  [unwired: 9 out]
          n148 = Close Reference(reference=w485) -> ()  [unwired: 1 in, 1 out]
        }
        frame Default {
        }
      }
      n149 = call-poly "DatabaseHand_Get.vi"("default value"=u32 0 ("unsigned 32bit integer"), "name"="expIDcounter" ("value"), "Database RefNum in"=w436) -> ("value"=w433:u32, "Database RefNum out"=w432:T1)  [unwired: 2 in, 5 out]
      n150 = call-poly "DatabaseHand_Get.vi"("name"="expIDbase" ("value"), "Database RefNum in"=w432) -> ("value"=w428:string, "Database RefNum out"=w431:T1)  [unwired: 3 in, 5 out]
      n151 = call-poly "DatabaseHand_Get.vi"("default value"=FALSE, "name"="autoexpID" ("value"), "Database RefNum in"=w431) -> ("value"=w427:bool)  [unwired: 2 in, 6 out]
      n152 = stacked-sequence {
        tunnel: w454 -> [w474 _]
        tunnel: w453 -> [w473 _]
        tunnel: w452 -> [w472 _]
        tunnel: w449 -> [w471 _]
        tunnel: w439 -> [w470 _]
        tunnel: w438 -> [w469 _]
        tunnel: w433 -> [_ w480]
        tunnel: w428 -> [_ w479]
        tunnel: w427 -> [_ w478]
        frame #0 {
          n153 = call "DHE_SaveImgparams.vi"("prefix"=w469, "sufix"=w470, "froot"=w471, "number"=w474, "basename"=w472, "dir"=w473) -> ()  [unwired: 6 out]
        }
        frame #1 {
          n154 = Select(t="on" ("value"), s=w478, f="off") -> (s? t:f=w475:string)
          n155 = call "DHE_SaveIDparams.vi"("autoid"=w475, "expidcounter"=w480, "expidbase"=w479) -> ()  [unwired: 9 out]
        }
      }
      n156 = call "DHE_SaveSyncMacro.vi"() -> ()  [unwired: 1 in, 11 out]
      n157 = call "DHE_SetImgState.vi"("DHE_ImgState"=T2."Idle") -> ()  [unwired: 9 out]
    }
    frame "INIT", "START" {
      n158 = Search 1D Array(1D array=w504, element="-force") -> (index of element=w509:i32)  [unwired: 1 out]
      n159 = call "DHE_GetStatus.vi"() -> ("DHE_Status"=w521:string)  [unwired: 9 out]
      n160 = Less Than 0?(x=w509) -> (x < 0?=w506:bool)
      n161 = Scan From String(format string="%s", input string=w521) -> (output 1=w519:string)  [unwired: 2 in, 4 out]
      n162 = Not Equal?(x=w519, y="NOT") -> (x != y?=w507:bool)
      n163 = Bundle By Name(cluster=w516, "status"=TRUE, "code"=-98, "source"="module already initialized") -> (w522:errorcluster)
      n164 = And(x=w507, y=w506) -> (x .and. y?=w508:bool)
      n165 = Select(t=w522, s=w508, f=w516) -> (s? t:f=w515:errorcluster)
      n166 = case shown="No Error" w515 {
        tunnel: w526 -> [w545 _]
        tunnel: [w537 w666] -> w514
        tunnel: w515 -> [w536 w666]
        tunnel: w505 -> [w532 _]
        tunnel: w504 -> [w531 _]
        tunnel: w503 -> [w530 _]
        tunnel: w502 -> [w529 _]
        tunnel: w501 -> [w528 w665]
        tunnel: [w527 w665] -> w500
        frame No Error {
          n167 = Current VI's Path() -> (path=w542:path)
          n168 = call "DHE_SetStatus.vi"("DHE_Status"="Initializing ...") -> ()  [unwired: 9 out]
          n169 = call "CMN_testpath.vi"("ModuleName"="ModuleName", "caller Path"=w542) -> ("error out"=w544:errorcluster, "ConfigFile"=w538:path)  [unwired: 1 in, 7 out]
          "ConfigFile" <- w538
          n170 = call "DatabaseHand_Create.vi"("Name"="DBS") -> ("Database RefNum out"=w534:T1)  [unwired: 1 in, 9 out]
          n171 = call "CMN_ConfigVals.vi"("error in (no error)"=w544, "Action"=enum16{"Read from File", "Write to File"}."Read from File", "ConfigVariables"="Config", "configuration file path"=w538) -> ("error out"=w539:errorcluster)  [unwired: 7 out]
          n172 = stacked-sequence {
            tunnel: w539 -> [_ _ _ _ _]
            tunnel: w536 -> [_ _ w611 _ w664]
            tunnel: w545 -> [w572 _ _ _ _]
            tunnel: w538 -> [_ w585 w598 _ _]
            tunnel: [_ _ _ _ w661] -> w537
            tunnel: w534 -> [w562 _ w591 w632 _]
            tunnel: w532 -> [_ _ _ _ w651]
            tunnel: w531 -> [_ _ _ w625 _]
            tunnel: w530 -> [_ _ _ _ w650]
            tunnel: w529 -> [_ _ _ _ w649]
            tunnel: w528 -> [_ _ _ _ w642]
            tunnel: [_ _ _ _ w641] -> w527
            frame #0 {
              n173 = Scan From String(format string="%s", input string=w572) -> (output 1=w570:string)  [unwired: 2 in, 4 out]
              n174 = Path To String(path="DHE_Aliasfile") -> (string=w549:string)
              n175 = call "DHE_TP.vi"("Command"="delete") -> ()  [unwired: 6 in, 9 out]
              n176 = case shown="\"\", \" \"" w570 {
                selector: w570 -> [w574 _]
                tunnel: "Init_file" -> [_ w575]
                tunnel: [w573 w575] -> w561
                frame Default {
                  n177 = String To Path(string=w574) -> (path=w573:path)
                }
                frame "", " " {
                }
              }
              n178 = call "DHE_InspectName.vi"("name in"=w549) -> ("name out"=w546:string)  [unwired: 10 out]
              n179 = call "DHE_SetDBS.vi"("DHE_DBSRef"=w562) -> ()  [unwired: 9 out]
              n180 = Current VI's Path() -> (path=w567:path)
              n181 = call "CMN_modinfo.vi"("caller path"=w567) -> ("INFO"=w566:string)  [unwired: 2 in, 8 out]
              n182 = call "DHE_Aliases.vi"("action"=enum16{"read from file", "find"}."read from file", "name in"=w546) -> ()  [unwired: 6 in, 4 out]
              n183 = Path To String(path=w561) -> (string=w559:string)
              n184 = call "DHE_InspectName.vi"("name in"=w559) -> ("name out"=w560:string)  [unwired: 10 out]
              n185 = String To Path(string=w560) -> (path=w558:path)
              n186 = call-poly "DatabaseHand_Set.vi"("group"="dhe", "name"="dhe_ver", "value"=w566, "Database RefNum in"=w562) -> ()  [unwired: 4 in, 4 out]
              n187 = call "DHE_SetConfigFile.vi"("DHE_ConfigFile"=w558) -> ()  [unwired: 9 out]
              n188 = Path To String(path="DHE_LogFile") -> (string=w552:string)
              n189 = call "DHE_SetLog.vi"("DHE_log"="log") -> ()  [unwired: 9 out]
              n190 = Path To String(path="DHE_InstLib") -> (string=w555:string)
              n191 = call "DHE_InspectName.vi"("name in"=w552) -> ("name out"=w551:string)  [unwired: 10 out]
              n192 = call "DHE_InspectName.vi"("name in"=w555) -> ("name out"=w556:string)  [unwired: 10 out]
              n193 = String To Path(string=w556) -> (path=w554:path)
              n194 = String To Path(string=w551) -> (path=w550:path)
              n195 = call "DHE_SetInstLibPath.vi"("DHE_InstLibPath"=w554) -> ()  [unwired: 9 out]
              n196 = call "DHE_SetLogFile.vi"("DHE_LogFile"=w550) -> ()  [unwired: 9 out]
            }
            frame #1 {
              n197 = Strip Path(path=w585) -> (stripped path=w584:path)  [unwired: 1 out]
              n198 = call "CMN_ReplaceName.vi"("name in"="FPAname") -> ("name out"=w577:string)  [unwired: 1 in, 9 out]
              n199 = call "DHE_GetInitCmdLine.vi"("fpa in"=w577) -> ("fpa out"=w576:string)  [unwired: 3 in, 7 out]
              n200 = call "DHE_SetFPAname.vi"("Path"=w584, "DHE_FPAname"=w576) -> ()  [unwired: 8 out]
              n201 = call "DHE_SetModifiers.vi"("DHE_Modifiers"="FPAmodifiers") -> ()  [unwired: 9 out]
              n202 = call "DHE_SetReadModeVar.vi"("DHE_ReadMode"="FPAreadmode") -> ()  [unwired: 9 out]
              n203 = call "DHE_InspectName.vi"("name in"="initmacro") -> ("name out"=w583:string)  [unwired: 10 out]
              n204 = call "DHE_InspectName.vi"("name in"="shutdownmacro") -> ("name out"=w582:string)  [unwired: 10 out]
              n205 = String To Path(string=w583) -> (path=w580:path)
              n206 = String To Path(string=w582) -> (path=w581:path)
              n207 = call "DHE_SetInitMacro.vi"("DHE_InitMacro"=w580) -> ()  [unwired: 9 out]
              n208 = call "DHE_SetShutdownMacro.vi"("DHE_InitMacro"=w581) -> ()  [unwired: 9 out]
              n209 = call "DHE_SetAppendID.vi"("DHE_appendid"="appendid") -> ()  [unwired: 9 out]
              n210 = call "DHE_SetAsyncExp.vi"("DHE_asyncexp"="expasync") -> ()  [unwired: 9 out]
            }
            frame #2 {
              # "overriden\n<-- if defined\non the DHE\nsubmodule"
              n211 = call "DHE_ReadTimingFromFile.vi"("configfile"=w598) -> ("timeout offset"=w594:i32)  [unwired: 1 in, 9 out]
              n212 = Greater Or Equal To 0?(x=w594) -> (x >= 0?=w595:bool)
              n213 = Path To String(path="TP_file") -> (string=w604:string)
              n214 = call "DHE_InspectName.vi"("name in"=w604) -> ("name out"=w605:string)  [unwired: 10 out]
              n215 = Select(t=w594, s=w595, f=30000) -> (s? t:f=→"timeout offset":i32)
              n216 = String To Path(string=w605) -> (path=w603:path)
              n217 = call "DHE_SetTPconfig.vi"("DHE_TPcfg"=w603) -> ()  [unwired: 9 out]
              n218 = call "DHE_ReadTPs.vi"("error in (no error)"=w611, "action"=DHE_TP_action."READ FROM FILE", "file path"=w603) -> ("error out"=w597:errorcluster)  [unwired: 4 in, 4 out]
              n219 = stacked-sequence {
                tunnel: w591 -> [w618]
                tunnel: w598 -> [w616]
                tunnel: w597 -> [_]
                frame #0 {
                  n220 = Path To String(path=w616) -> (string=w614:string)
                  n221 = call "DHE_InspectName.vi"("name in"=w614) -> ("name out"=w615:string)  [unwired: 10 out]
                  n222 = String To Path(string=w615) -> (path=w613:path)
                  n223 = call "DHE_template2keys.vi"("Action"=T7."read from file", "file"=w613) -> ("HdrInfo"=w619:string[][])  [unwired: 2 in, 7 out]
                  n224 = call-poly "DatabaseHand_Set.vi"("group"="HDR", "name"="DHEINFO", "value"=w619, "Database RefNum in"=w618) -> ()  [unwired: 4 in, 4 out]
                }
              }
              n225 = Path To String(path="DHE_MacroDir") -> (string=w608:string)
              n226 = call "DHE_InspectName.vi"("name in"=w608) -> ("name out"=w609:string)  [unwired: 10 out]
              n227 = Path To String(path="Algors_file") -> (string=w600:string)
              n228 = String To Path(string=w609) -> (path=w607:path)
              n229 = call "DHE_InspectName.vi"("name in"=w600) -> ("name out"=w602:string)  [unwired: 10 out]
              n230 = call "DHE_SetMacroDir.vi"("DHE_MacroDir"=w607) -> ()  [unwired: 9 out]
              n231 = String To Path(string=w602) -> (path=w599:path)
              n232 = call "DHE_SetAlgorsFile.vi"("DHE_AlgorsFile"=w599) -> ()  [unwired: 9 out]
              n233 = call "CMN_Algors.vi"("file"=w599, "action"=enum16{"convert", "read from file", "get"}."read from file") -> ()  [unwired: 3 in, 6 out]
            }
            frame #3 {
              w630 = "dhe_init" ("name")
              n234 = call-poly "DatabaseHand_Get.vi"("name"=w630, "Database RefNum in"=w632) -> ("error out"=w631:errorcluster, "Database RefNum out"=w627:T1)  [unwired: 3 in, 5 out]
              n235 = case shown="Error" w631 {
                tunnel: [TRUE w634] -> w629
                frame No Error {
                }
                frame Error {
                  n236 = property class="App"() -> ("Application:Command Line Arguments"=w637:string[])  [unwired: 2 in, 2 out]
                  n237 = Search 1D Array(1D array=w637, element="-no_hdwinit") -> (index of element=w635:i32)  [unwired: 1 out]
                  n238 = Less Than 0?(x=w635) -> (x < 0?=w634:bool)
                }
              }
              n239 = Search 1D Array(1D array=w625, element="-no_hdwinit") -> (index of element=w624:i32)  [unwired: 1 out]
              n240 = Less Than 0?(x=w624) -> (x < 0?=w623:bool)
              n241 = And(x=w623, y=w629) -> (x .and. y?=w628:bool)
              n242 = call-poly "DatabaseHand_Set.vi"("name"=w630, "value"=w628, "Database RefNum in"=w627) -> ()  [unwired: 5 in, 4 out]
              n243 = call "DHE_SetExtShutter.vi"("Ext_Shutter"="extshut") -> ()  [unwired: 9 out]
            }
            frame #4 {
              w648 = u16 3 items=["command", "imediateReply", "Callback Reply", "Information", "none"] ("type")
              # "^\n      |\noverriden\nif defined\non the DHE\nsubmodule"
              n244 = Multiply(x="initimeout", y=1000) -> (x*y=w638:i32)
              n245 = Greater Than 0?(x="initimeout") -> (x > 0?=w643:bool)
              n246 = call "DHE_SyncImage.vi"() -> ("cmds2exec"=w663:string[])  [unwired: 4 in, 7 out]
              n247 = Select(t=w638, s=w643, f=w642) -> (s? t:f=w641:i32)
              n248 = call "DHE_LoadDHEModule.vi"("ModuleName"="DHE_Mod", "modpath"=w651) -> ("error out"=w644:errorcluster)  [unwired: 1 in, 8 out]
              n249 = call "DHE_SetArtifPatterns.vi"("DHE_ArtifPatterns"="artifpatterns") -> ()  [unwired: 9 out]
              n250 = call "DHE_CheckBusy.vi"("error in (no error)"=w664) -> ("error out"=w662:errorcluster)  [unwired: 2 in, 8 out]
              n251 = call "DHE_SetCommandToExecute.vi"("DHE_Commands2Exec"=w663) -> ()  [unwired: 9 out]
              n252 = Unbundle By Name(w644) -> ("code"=w645:i32)
              n253 = Merge Errors(w662, w644) -> (w661:errorcluster)
              n254 = Path To String(path="DHE_REGfile") -> (string=w653:string)
              n255 = call "DHE_InspectName.vi"("name in"=w653) -> ("name out"=w654:string)  [unwired: 10 out]
              n256 = Path To String(path="DHE_DACfile") -> (string=w656:string)
              n257 = Format Into String(format string="Loading module %s %d" ("string"), "DHE_Mod", w645) -> ()  [unwired: 2 in, 2 out]
              n258 = String To Path(string=w654) -> (path=w652:path)
              n259 = call "DHE_InspectName.vi"("name in"=w656) -> ("name out"=w658:string)  [unwired: 10 out]
              n260 = call "DHE_SetREGsFile.vi"("DHE_REGsFile"=w652) -> ()  [unwired: 9 out]
              n261 = call "CMN_ToServerLogQ.vi"("Log"=w649, "file"=w650, "type"=w648) -> ()  [unwired: 3 in, 5 out]
              n262 = String To Path(string=w658) -> (path=w657:path)
              n263 = call "DHE_SetDACsFile.vi"("DHE_DACsFile"=w657) -> ()  [unwired: 9 out]
            }
          }
        }
        frame Error {
        }
      }
      n264 = Unbundle By Name(w514) -> ("source"=w517:string)
      n265 = Format Into String(format string="%s %d", "OK", w500) -> (resulting string=w511:string)  [unwired: 2 in, 1 out]
    }
    frame "ASYNC" {
      n266 = Scan From String(format string="%s", input string=w670) -> (remaining string=w675:string, output 1=w677:string)  [unwired: 2 in, 3 out]
      n267 = To Upper Case(1:w677) -> (0:w676:string)
      n268 = case shown="\"GET\", \"PARAMS\"" w676 {
        selector: w676 -> [_ _ _ _ _ _ _ _ _ w761 _]
        tunnel: [enum16{"ERROR", "WARNING", "INFO", "CHANGED"}."INFO" ("type") enum16{"ERROR", "WARNING", "INFO", "CHANGED"}."INFO" ("type") enum16{"ERROR", "WARNING", "INFO", "CHANGED"}."INFO" ("type") enum16{"ERROR", "WARNING", "INFO", "CHANGED"}."INFO" ("type") enum16{"ERROR", "WARNING", "INFO", "CHANGED"}."INFO" ("type") enum16{"ERROR", "WARNING", "INFO", "CHANGED"}."INFO" ("type") enum16{"ERROR", "WARNING", "INFO", "CHANGED"}."INFO" ("type") enum16{"ERROR", "WARNING", "INFO", "CHANGED"}."INFO" ("type") enum16{"ERROR", "WARNING", "INFO", "CHANGED"}."INFO" ("type") w765 enum16{"ERROR", "WARNING", "INFO", "CHANGED"}."INFO" ("type")] -> w672
        tunnel: w675 -> [_ w709 _ _ _ _ _ _ w752 w760 _]
        tunnel: w674 -> [_ _ _ _ w728 _ _ _ _ w763 _]
        tunnel: ["" "" "" "" "" "" "" "" "" w762 "TESTING ASYNC CHANNEL" ("trimmed string")] -> w671
        tunnel: w670 -> [_ _ _ _ _ _ _ _ _ w758 _]
        tunnel: [FALSE ("asyncch") FALSE ("asyncch") FALSE ("asyncch") FALSE ("asyncch") FALSE ("asyncch") FALSE ("asyncch") FALSE ("asyncch") FALSE ("asyncch") FALSE ("asyncch") w756 w785] -> w668
        tunnel: [w687 "DONE" "DONE" "DONE" w724 "DONE" "DONE" "DONE" "DONE" "DONE" "DONE"] -> w667
        frame "GET", "PARAMS" {
          n269 = call "DHE_asyncvarsMgr.vi"("action"=T8."get") -> ("statusch"=w685:bool, "enabled"=w696:bool, "names"=w697:string[])  [unwired: 3 in, 5 out]
          n270 = Select(t="using_status_ch" ("resulting string"), s=w685, f="using_async_ch" ("resulting string")) -> (s? t:f=w686:string)
          n271 = Format Into String(format string="enabled= %s, %s, \\nVars: ", w696, w686) -> (resulting string=w694:string)  [unwired: 2 in, 1 out]
          n272 = for {
            tunnel: w697 -> [w703] mode=indexing
            shift-right: [w702] -> w693
            shift-left: w694 -> [w704]
            n273 = Concatenate Strings(w704, w703, ", " ("string")) -> (w702:string)
          }
          n274 = call <vilib>:"Trim Whitespace.vi"("string"=w693) -> ("trimmed string"=w691:string)  [unwired: 1 in]
          n275 = Reverse String(1:w691) -> (0:w690:string)
          n276 = String Subset(string=w690, offset (0)=1) -> (substring=w688:string)  [unwired: 1 out]
          n277 = Reverse String(1:w688) -> (0:w687:string)
        }
        frame "ADD" {
          n278 = call <vilib>:"Trim Whitespace.vi"("string"=w709) -> ("trimmed string"=w708:string)  [unwired: 1 in]
          n279 = call "DHE_asyncvarsMgr.vi"("action"=T8."add", "var"=w708) -> ()  [unwired: 2 in, 8 out]
        }
        frame "ALL" {
          n280 = call "DHE_asyncvarsMgr.vi"("action"=T8."send_all") -> ()  [unwired: 3 in, 8 out]
        }
        frame "0", "DISABLE", "FALSE", "OFF" {
          n281 = call "DHE_asyncvarsMgr.vi"("action"=T8."send_off") -> ()  [unwired: 3 in, 8 out]
        }
        frame "STATCH", "USESTAT", "USE_STAT" {
          n282 = call-poly "DatabaseHand_Get.vi"("default value"=FALSE, "name"="status_present", "Database RefNum in"=w728) -> ("value"=w722:bool)  [unwired: 2 in, 6 out]
          n283 = case shown="True" w722 {
            frame False {
            }
            frame True {
              n284 = call "DHE_asyncvarsMgr.vi"("action"=T8."use_stat") -> ()  [unwired: 3 in, 8 out]
            }
          }
          n285 = Select(t="DONE", s=w722, f="ERROR STATUS module is NOT present") -> (s? t:f=w724:string)
        }
        frame "ASYNCCH", "USEASYNC", "USE_ASYNC" {
          n286 = call "DHE_asyncvarsMgr.vi"("action"=T8."use_async") -> ()  [unwired: 3 in, 8 out]
        }
        frame "1", "ENABLE", "ON", "TRUE", "YES" {
          n287 = call "DHE_asyncvarsMgr.vi"("action"=T8."send_on") -> ()  [unwired: 3 in, 8 out]
        }
        frame "CLEAN" {
          n288 = call "DHE_asyncvarsMgr.vi"("action"=T8."clean") -> ()  [unwired: 3 in, 8 out]
        }
        frame "DELETE" {
          n289 = call <vilib>:"Trim Whitespace.vi"("string"=w752) -> ("trimmed string"=w751:string)  [unwired: 1 in]
          n290 = call "DHE_asyncvarsMgr.vi"("action"=T8."delete", "var"=w751) -> ()  [unwired: 2 in, 8 out]
        }
        frame "SEND", Default {
          n291 = case shown="Default" w761 {
            tunnel: w760 -> [_ w770]
            tunnel: [w769 w770] -> w759
            tunnel: w758 -> [w769 _]
            frame Default {
            }
            frame "SEND" {
            }
          }
          n292 = Scan From String(format string="%s", input string=w759) -> (remaining string=w764:string, output 1=w767:string)  [unwired: 2 in, 3 out]
          n293 = To Upper Case(1:w767) -> (0:w766:string)
          n294 = case shown="Default" w766 {
            tunnel: [enum16{"ERROR", "WARNING", "INFO", "CHANGED"}."INFO" ("type") enum16{"ERROR", "WARNING", "INFO", "CHANGED"}."INFO" ("type") enum16{"ERROR", "WARNING", "INFO", "CHANGED"}."CHANGED" ("type")] -> w765
            tunnel: w764 -> [w772 _ _]
            tunnel: [w771 w775 w779] -> w762
            tunnel: w763 -> [_ _ w778]
            tunnel: w759 -> [_ w774 _]
            frame "INFO", "MSG" {
              n295 = call <vilib>:"Trim Whitespace.vi"("string"=w772) -> ("trimmed string"=w771:string)  [unwired: 1 in]
            }
            frame Default {
              n296 = call <vilib>:"Trim Whitespace.vi"("string"=w774) -> ("trimmed string"=w775:string)  [unwired: 1 in]
            }
            frame "UPDATE" {
              n297 = call "DHE_GetProgress.vi"("Databse Ref"=w778) -> ("progress"=w777:string)  [unwired: 1 in, 9 out]
              n298 = Concatenate Strings("IMVARS " ("string"), w777) -> (w779:string)
            }
          }
          n299 = call "DHE_asyncvarsMgr.vi"("action"=T8."get") -> ("statusch"=w756:bool)  [unwired: 3 in, 7 out]
        }
        frame "TEST" {
          n300 = call "DHE_asyncvarsMgr.vi"("action"=T8."get") -> ("statusch"=w785:bool)  [unwired: 3 in, 7 out]
        }
      }
      n301 = case shown="True" w668 {
        tunnel: w672 -> [w681 _]
        tunnel: w671 -> [w680 w682]
        frame False {
          n302 = call "DHE_SendAsync.vi"("type"=w681, "Message"=w680) -> ()  [unwired: 10 out]
        }
        frame True {
          n303 = call "DHE_SendStat.vi"("Message"=w682) -> ()  [unwired: 11 out]
        }
      }
    }
    frame "VERSION" {
      n304 = Search 1D Array(1D array=w800, element="-full") -> (index of element=w798:i32)  [unwired: 1 out]
      n305 = Greater Or Equal To 0?(x=w798) -> (x >= 0?=w788:bool)
      n306 = Current VI's Path() -> (path=w797:path)
      n307 = call "CMN_modinfo.vi"("error in (no error)"=w796, "full"=w788, "caller path"=w797) -> ("error out"=w795:errorcluster, "INFO"=w790:string)  [unwired: 7 out]
      n308 = call "DHE_version.vi"("fd in"=w793, "full"=w788, "error in (no error)"=w795) -> ("version"=w791:string, "error out"=w794:errorcluster)  [unwired: 11 out]
      n309 = Concatenate Strings(w790, "\n", w791) -> (w789:string)
    }
    frame "ALIAS" {
      n310 = Scan From String(format string="%s", input string=w801) -> (remaining string=w802:string, output 1=w804:string)  [unwired: 3 in, 2 out]
      n311 = case shown="Default" w804 {
        tunnel: [w808 w812 w814] -> w803
        tunnel: w802 -> [w810 _ _]
        frame "add", "set" {
          n312 = call <vilib>:"Trim Whitespace.vi"("string"=w810) -> ("trimmed string"=w809:string)  [unwired: 1 in]
          n313 = call "DHE_Aliases.vi"("action"=T9."add", "name in"=w809) -> ("name out"=w808:string)  [unwired: 6 in, 3 out]
        }
        frame "clear", "clearall" {
          n314 = call "DHE_Aliases.vi"("action"=T9."clear ") -> ("name out"=w812:string)  [unwired: 7 in, 3 out]
        }
        frame Default {
          n315 = call "DHE_Aliases.vi"("action"=T9."get") -> ("name out"=w814:string)  [unwired: 7 in, 3 out]
        }
      }
    }
    frame "DBS" {
      n316 = Scan From String(format string="%s", input string=w817) -> (remaining string=w818:string, output 1=w820:string)  [unwired: 3 in, 2 out]
      n317 = case shown="\"set\"" w820 {
        tunnel: [w825 w840 "ERROR <get | set>" ("response")] -> w819
        tunnel: w818 -> [w831 w844 _]
        tunnel: w816 -> [w824 w845 _]
        frame "set" {
          n318 = Scan From String(format string="%s %s", input string=w831) -> (output 1=w828:string, output 2=w827:string)  [unwired: 4 in, 3 out]
          n319 = call-poly "DatabaseHand_Get.vi"("name"=w828, "Database RefNum in"=w824) -> ("error out"=w829:errorcluster, "type"=w826:string)  [unwired: 3 in, 5 out]
          n320 = case shown="No Error" w829 {
            tunnel: w824 -> [w837 _]
            tunnel: w828 -> [w836 _]
            tunnel: w827 -> [w835 _]
            tunnel: w826 -> [w834 _]
            tunnel: [w833 "ERROR unknow var" ("response")] -> w825
            frame No Error {
              n321 = call "DHE_DBS_SetByType.vi"("queue?"=FALSE, "type"=w834, "value"=w835, "name"=w836, "Database RefNum"=w837) -> ("response"=w833:string)  [unwired: 6 in]
            }
            frame Error {
            }
          }
        }
        frame "get" {
          n322 = Scan From String(format string="%s", input string=w844) -> (output 1=w842:string)  [unwired: 3 in, 3 out]
          n323 = call-poly "DatabaseHand_Get.vi"("name"=w842, "Database RefNum in"=w845) -> ("error out"=w841:errorcluster, "value"=w839:string)  [unwired: 3 in, 5 out]
          n324 = case shown="Error" w841 {
            tunnel: [w846 "ERROR unknow var" ("response")] -> w840
            tunnel: w839 -> [w846 _]
            frame No Error {
            }
            frame Error {
            }
          }
        }
        frame Default {
        }
      }
    }
  }
  "message" <- w5
  "OK message" <- w22
  "TimeOut out" <- w10
  n325 = call "CMN_ToServerLogQ.vi"("error in (no error)"=w4, "Log"="Log", "file"=w3, "string"=w5, "type"=w6) -> ()  [unwired: 1 in, 5 out]
  n326 = case shown="No Error" w15 {
    selector: w15 -> [w852 w856]
    tunnel: [w849 w856] -> w14
    frame No Error {
      n327 = Unbundle By Name(w852) -> ("code"=w855:i32)
      n328 = Bundle By Name(cluster=w852, "code"=0) -> (w851:errorcluster)
      n329 = Not Equal?(x=w855, y=4476750) -> (x != y?=w853:bool)
      n330 = Select(t=w852, s=w853, f=w851) -> (s? t:f=w849:errorcluster)
    }
    frame Error {
    }
  }
  "error out" <- w14
